vi "Begin.vi"(11 "Image Size":T1=enum."160x120") -> (0 "error out":errorcluster)   [LabVIEW 2012]
doc: "Called before other user functions, this VI is expected to open initial I/O refnums, load in file data, and do all program initialization. Notice that the <B>error out</B> terminal is simply used for data flow. Wiring it to other structures or subVIs ensures that this VI runs first."
uses:
  <vilib>/Rock Robotics/WPI/Camera/WPI_CameraImageSize.ctl
  <vilib>/Rock Robotics/WPI/SafetyOutput/WPI_SafetyOutputConfigMenu.ctl
  <vilib>/Rock Robotics/WPI/DriverStation/WPI_DriverStationRobotMode2.ctl
  <vilib>/Rock Robotics/WPI/Joystick/WPI_JoystickDeviceEnum.ctl
  <vilib>/Rock Robotics/SystemInterfaces/DIO/FPGA_DIOPWMChannel.ctl
  <vilib>/Rock Robotics/WPI/Solenoid/WPI_SolenoidChannel.ctl
  <vilib>/Rock Robotics/SystemInterfaces/DIO/FPGA_DIOChannel.ctl
  <vilib>/Rock Robotics/SystemInterfaces/DIO/FPGA_DIORelayChannel.ctl
  <vilib>/Rock Robotics/SystemInterfaces/AI/FPGA_AIChannel.ctl
  Robot Global Data.vi
  <vilib>/Rock Robotics/WPI/MotorControl/WPI_MotorControlOpen Talon.vi
  <vilib>/Rock Robotics/WPI/RobotDrive/WPI_RobotDriveOpen4MotorWithTalon.vi
  <vilib>/Rock Robotics/WPI/Solenoid/WPI_SolenoidOpenDouble.vi
  <vilib>/Rock Robotics/WPI/MotorControl/WPI_MotorControlOpen Victor.vi
  <vilib>/Rock Robotics/WPI/Counter/WPI_CounterDigitalInputToDigitalSource.vi
  <vilib>/Rock Robotics/WPI/Compressor/WPI_CompressorGetSetRefNum.vi
  <vilib>/Rock Robotics/WPI/Camera/WPI_CameraWhite Balance Values.ctl
  <vilib>/Rock Robotics/WPI/Camera/WPI_CameraExposure Values.ctl
  <vilib>/Rock Robotics/WPI/Camera/WPI_CameraFrameRate.ctl
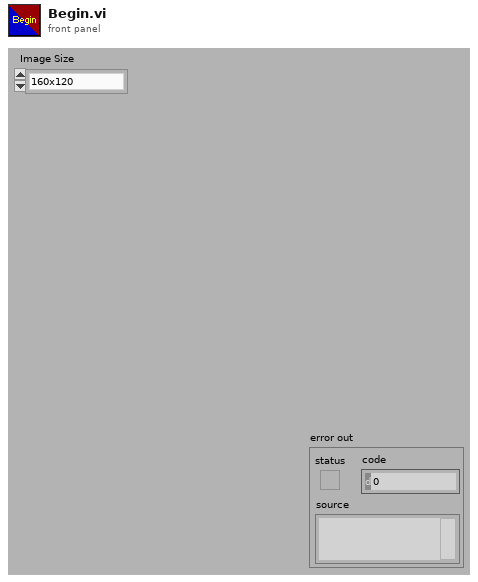
[diagram p1: front panel]
types:
  T1 = typedef "WPI_CameraImageSize.ctl" = enum16{"640x480", "320x240", "160x120"}
  T2 = typedef "FPGA_DIOChannel.ctl" = enum8{"DIO 1", "DIO 2", "DIO 3", "DIO 4", "DIO 5", "DIO 6", "DIO 7", "DIO 8", "DIO 9", "DIO 10", "DIO 11", "DIO 12", "DIO 13", "DIO 14", "Invalid"}
  T3 = typedef "WPI_SolenoidChannel.ctl" = enum8{"Solenoid 1", "Solenoid 2", "Solenoid 3", "Solenoid 4", "Solenoid 5", "Solenoid 6", "Solenoid 7", "Solenoid 8", "Invalid"}
  T4 = typedef "FPGA_AIChannel.ctl" = enum8{"AI 1", "AI 2", "AI 3", "AI 4", "AI 5", "AI 6", "AI 7", "AI 8", "Invalid"}
  T5 = typedef "FPGA_DIOPWMChannel.ctl" = enum8{"PWM 1", "PWM 2", "PWM 3", "PWM 4", "PWM 5", "PWM 6", "PWM 7", "PWM 8", "PWM 9", "PWM 10", "Invalid"}
  T6 = typedef "FPGA_DIORelayChannel.ctl" = enum8{"Relay 1", "Relay 2", "Relay 3", "Relay 4", "Relay 5", "Relay 6", "Relay 7", "Relay 8", "Invalid"}
  T7 = typedef "WPI_JoystickDeviceEnum.ctl" = enum16{"USB 1", "USB 2", "USB 3", "USB 4", "Kinect 1", "Kinect 2"}
  T8 = typedef "WPI_DriverStationRobotMode2.ctl" = enum16{"Autonomous Disabled", "Autonomous Enabled", "Teleop Disabled", "Teleop Enabled", "Timeout", "Finish", "Test Disabled", "Test Enabled"}
  T9 = typedef "WPI_SafetyOutputConfigMenu.ctl" = enum16{"Enable", "Disable"}
  T10 = typedef "WPI_CameraFrameRate.ctl" = u32
  T11 = typedef "WPI_CameraExposure Values.ctl" = enum16{"Auto", "Flicker-free 50 Hz", "Flicker-free 60 Hz", "Hold current"}
  T12 = typedef "WPI_CameraWhite Balance Values.ctl" = enum16{"Auto", "Fixed indoor", "Fixed outdoor 1", "Fixed outdoor 2", "Fixed fluorescent 1", "Fixed fluorescent 2", "Hold current"}
  T13 = typedef "WPI_CameraDevRef.ctl" = cluster{"Camera Address":string, "CameraStatus":errorcluster, "Acquire Image Notifier":refnum<notifier>}
  T14 = typedef "WPI_RobotDriveDevRef.ctl" = cluster{"DevStatus":errorcluster, "Motors[]":T15[], "Square Inputs":bool, "Max Output":dbl, "Isochronous":bool}
  T15 = typedef "WPI_MotorControlDeviceRef.ctl" = cluster{"DeviceStatus":errorcluster, "Type":enum16{"PWM", "CAN"}, "PWM":cluster{"Digital Module":T16, "PWM Channel":T5, "DeadBand":T17}, "CAN":cluster{"Device Number":u8, "Control Mode":T18, "Semaphore":T19, "Max Vout":dbl}, "Invert":bool, "TransformRef":T20, "InvTransformRef":T20}
  T16 = typedef "FPGA_TypedefDigitalModule.ctl" = enum16{"Digital Module 1", "Digital Module 2"}
  T17 = typedef "WPI_PWMDeadband.ctl" = cluster{"Name":string, "maxPositivePwm":i32, "minPositivePwm":i32, "centerPwm":i32, "maxNegativePwm":i32, "minNegativePwm":i32, "angularRange":u16}
  T18 = typedef "WPI_CANJaguar_ControlMode.ctl" = enum8{"Percent VBus", "Current", "Speed", "Position", "Voltage"}
  T19 = typedef "Semaphore RefNum" = refnum<k1>
  T20 = typedef "WPI_PWMTransform_ConPane.ctl" = refnum<vi>
  T21 = typedef "WPI_DigitalInputDevRef.ctl" = cluster{"DevStatus":errorcluster, "DIO Channel":T2, "Digital Module":T16}
  T22 = typedef "WPI_SolenoidDevRef.ctl" = cluster{"DevStatus":errorcluster, "Solenoid Module":T23, "Forward Solenoid Channel":T3, "Reverse Solenoid Channel":T3}
  T23 = typedef "FPGA_TypedefSolenoidModule.ctl" = enum16{"Solenoid Module 1", "Solenoid Module 2"}
  T24 = typedef "WPI_CompressorDevRef.ctl" = cluster{"DevStatus":errorcluster, "DigitalInputDevRef":T21, "RelayDevRef":T25}
  T25 = typedef "WPI_RelayDevRef.ctl" = cluster{"DevStatus":errorcluster, "Relay Channel":T6, "Digital Module":T16, "Relay Direction":T26}
  T26 = typedef "WPI_RelayDirection.ctl" = enum16{"Both directions", "Forward only", "Reverse only"}
  T27 = typedef "WPI_JoystickDevRef.ctl" = cluster{"Device":T7}
  T28 = typedef "WPI_AnalogChannelDevRef.ctl" = cluster{"DevStatus":errorcluster, "Analog Module":T29, "Analog Channel":T4}
  T29 = typedef "FPGA_TypedefAnalogModule.ctl" = enum16{"Analog Module 1", "Analog Module 2"}
  T30 = typedef "FPGA_CounterEncoderSourceConvertionLVSourceType.ctl" = cluster{"DevStatus":errorcluster, "AnalogTriggerMode?":bool, "DigitalMode":cluster{"Digital Module":T16, "DIO Channel":T31}, "AnalogTriggerMode":cluster{"AnalogTriggerIndex":T32, "OutputType":T33}}
  T31 = typedef "FPGA_DIODigitalSourceChannel.ctl" = enum8{"DIO 1", "DIO 2", "DIO 3", "DIO 4", "DIO 5", "DIO 6", "DIO 7", "DIO 8", "DIO 9", "DIO 10", "DIO 11", "DIO 12", "DIO 13", "DIO 14", "Disabled"}
  T32 = typedef "FPGA_AnalogTriggerIndex.ctl" = enum8{"Trig 0", "Trig 1", "Trig 2", "Trig 3", "Trig 4", "Trig 5", "Trig 6", "Trig 7", "Invalid"}
  T33 = typedef "FPGA_AnalogTriggerOutType.ctl" = enum16{"InWindow", "TriggerState", "Rising", "Falling"}
  T34 = typedef "WPI_EncoderDevRef.ctl" = cluster{"DevStatus":errorcluster, "EncoderIndex":T35, "CounterIndex":T36, "DistancePerCount":dbl, "Decoding Type":T37}
  T35 = typedef "FPGA_EncoderIdx.ctl" = enum8{"Enc 0", "Enc 1", "Enc 2", "Enc 3", "Invalid"}
  T36 = typedef "FPGA_CounterCtrSystemIndex.ctl" = enum8{"Ctr 0", "Ctr 1", "Ctr 2", "Ctr 3", "Ctr 4", "Ctr 5", "Ctr 6", "Ctr 7", "Invalid"}
  T37 = typedef "WPI_EncoderType.ctl" = enum16{"1x", "2x", "4x"}
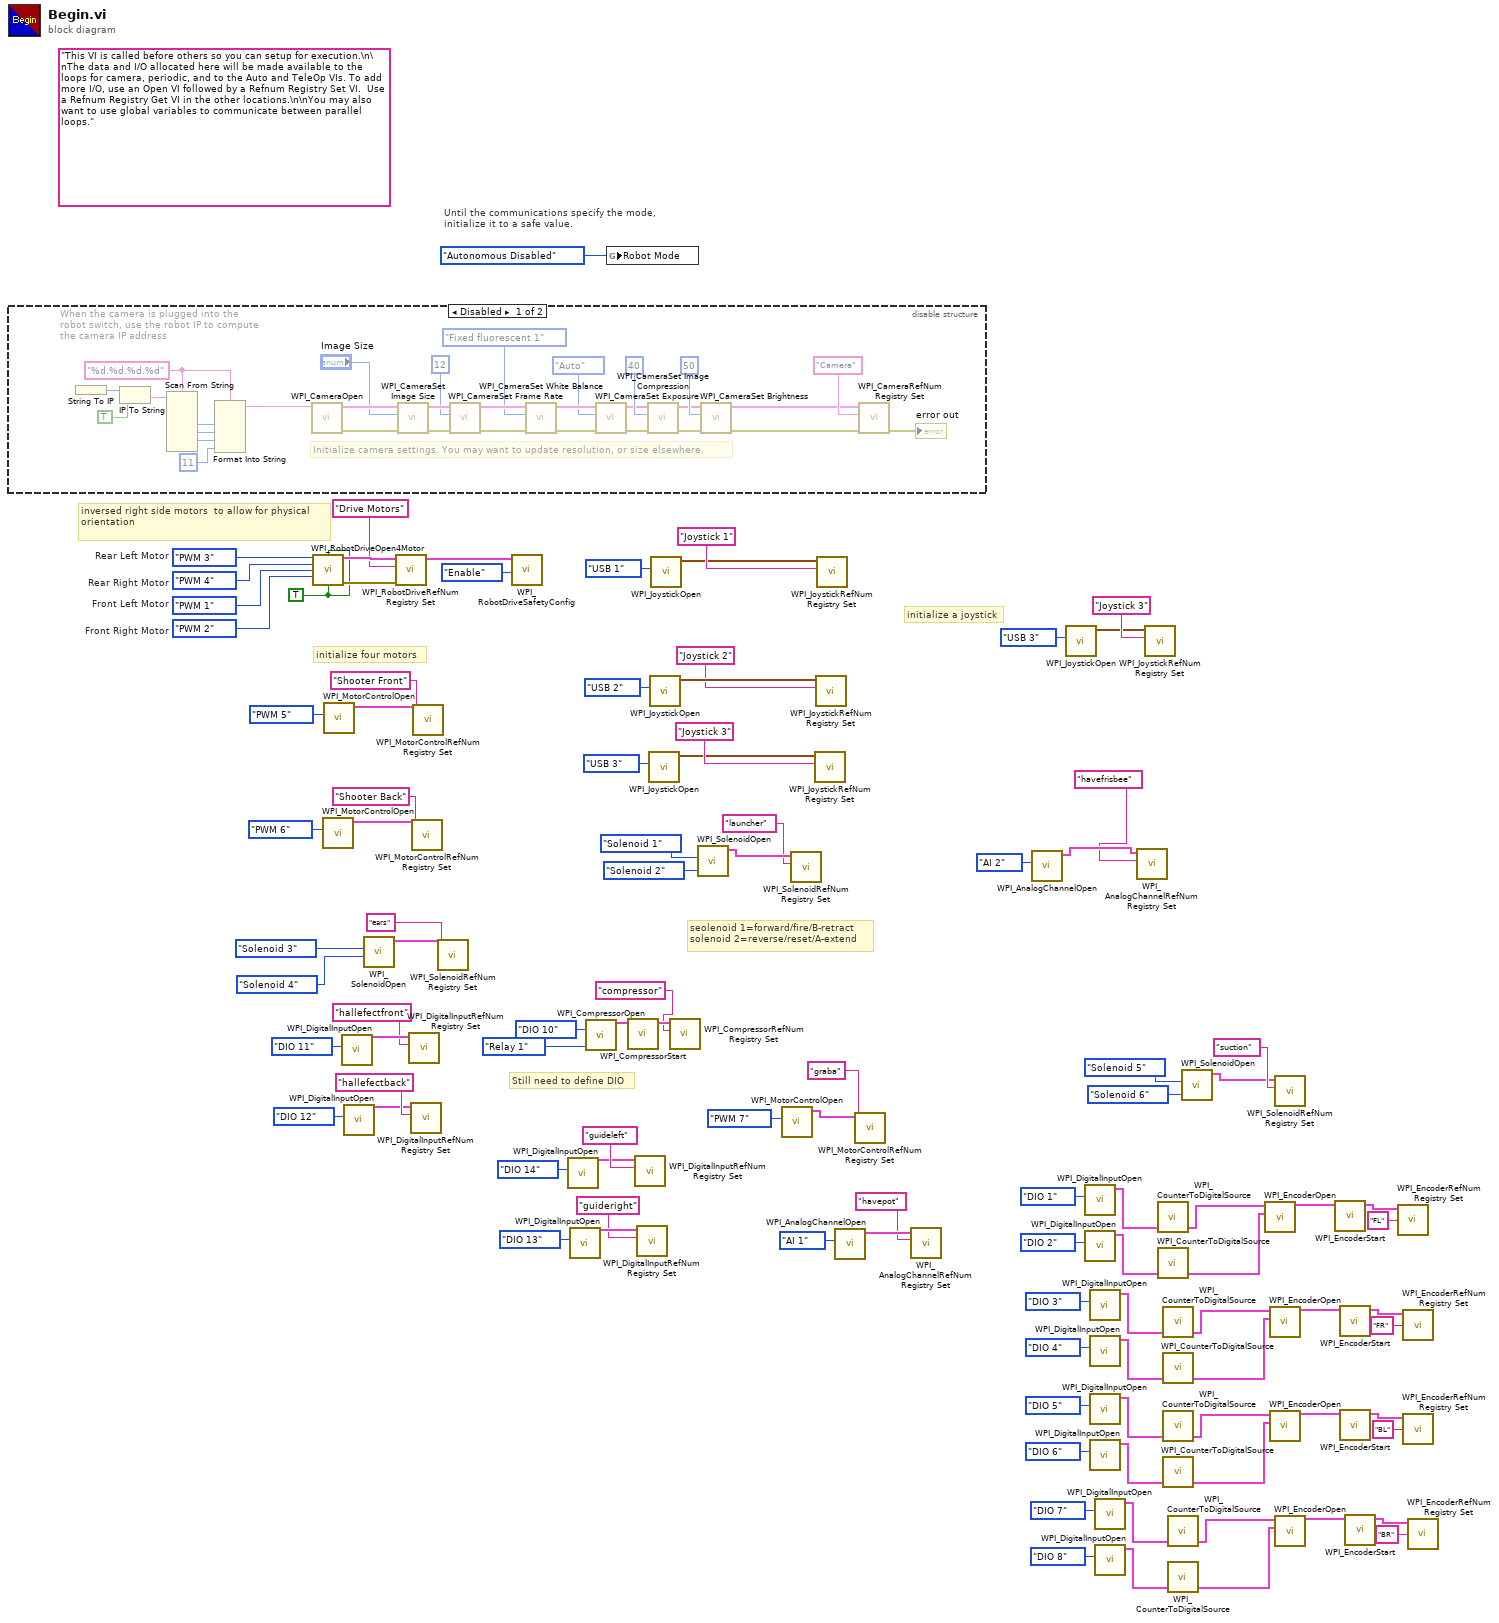
[diagram p0: block diagram]
diagram:
  w84 = TRUE ("Front Right Motor Inverted")
  w91 = FPGA_DIOPWMChannel."PWM 2"  # Front Right Motor
  w92 = FPGA_DIOPWMChannel."PWM 1"  # Front Left Motor
  w93 = FPGA_DIOPWMChannel."PWM 4"  # Rear Right Motor
  w94 = FPGA_DIOPWMChannel."PWM 3"  # Rear Left Motor
  (unwired) "This VI is called before others so you can setup for execution.\n\nThe data and I/O allocated here will be made available to the loops for camera, periodic, and to the Auto and TeleOp VIs. To add more I/O, use an Open VI followed by a Refnum Registry Set VI.  Use a Refnum Registry Get VI in the other locations.\n\nYou may also want to use global variables to communicate between parallel loops."
  # "Still need to define DIO"
  # "seolenoid 1=forward/fire/B-retract\nsolenoid 2=reverse/reset/A-extend"
  # "initialize a joystick"
  # "inversed right side motors  to allow for physical orientation"
  # "Until the communications specify the mode,\ninitialize it to a safe value."
  # "initialize four motors"
  n1 = disable-structure shown="Disabled" {
    frame Disabled {
      w106 = "%d.%d.%d.%d" ("format string")
      # "When the camera is plugged into the\nrobot switch, use the robot IP to compute\nthe camera IP address"
      # "Initialize camera settings. You may want to update resolution, or size elsewhere."
      n2 = String To IP() -> (0:w113:u32)  [unwired: 1 in]
      n3 = IP To String(1:TRUE ("dot notation? (F)"), 2:w113) -> (0:w111:string)
      n4 = Scan From String(format string=w106, input string=w111) -> (output 1=w110:i32, output 2=w109:i32, output 3=w108:i32)  [unwired: 7 in, 3 out]
      n5 = Format Into String(format string=w106, w110, w109, w108, 11 ("Compression")) -> (resulting string=w105:string)  [unwired: 2 in, 1 out]
      n6 = call <vilib>:"WPI_CameraOpen.vi"("Camera Address"=w105) -> ("error out"=w125:errorcluster, "CameraDevRef"=w126:T13)  [unwired: 1 in, 8 out]
      n7 = call <vilib>:"WPI_CameraSet Image Size.vi"("error in (no error)"=w125, "Image Size"="Image Size", "CameraDevRef"=w126) -> ("error out"=w124:errorcluster, "CameraDevRef Out"=w127:T13)  [unwired: 7 out]
      n8 = call <vilib>:"WPI_CameraSet Frame Rate.vi"("error in (no error)"=w124, "Frame Rate (fps)"=T10 12, "CameraDevRef"=w127) -> ("error out"=w123:errorcluster, "CameraDevRef Out"=w129:T13)  [unwired: 7 out]
      n9 = call <vilib>:"WPI_CameraSet White Balance.vi"("error in (no error)"=w123, "White Balance"=WPI_CameraWhite_Balance_Values."Fixed fluorescent 1", "CameraDevRef"=w129) -> ("error out"=w122:errorcluster, "CameraDevRef Out"=w128:T13)  [unwired: 7 out]
      n10 = call <vilib>:"WPI_CameraSet Exposure.vi"("error in (no error)"=w122, "Exposure"=WPI_CameraExposure_Values."Auto", "CameraDevRef"=w128) -> ("error out"=w121:errorcluster, "CameraDevRef Out"=w131:T13)  [unwired: 7 out]
      n11 = call <vilib>:"WPI_CameraSet Image Compression.vi"("error in (no error)"=w121, "Compression"=40, "CameraDevRef"=w131) -> ("error out"=w120:errorcluster, "CameraDevRef Out"=w130:T13)  [unwired: 7 out]
      n12 = call <vilib>:"WPI_CameraSet Brightness.vi"("error in (no error)"=w120, "Brightness"=50, "CameraDevRef"=w130) -> ("error out"=w118:errorcluster, "CameraDevRef Out"=w119:T13)  [unwired: 7 out]
      n13 = call <vilib>:"WPI_CameraRefNum Registry Set.vi"("error in (no error)"=w118, "refnum name"="Camera", "CameraDevRef"=w119) -> ("error out"=→"error out":errorcluster)  [unwired: 8 out]
    }
    frame Enabled {
    }
  }
  n14 = call-poly <vilib>:"WPI_RobotDriveOpen4Motor.vi"("Rear Left Motor"=w94, "Rear Right Motor Inverted"=w84, "Rear Right Motor"=w93, "Front Left Motor"=w92, "Front Right Motor"=w91, "Front Right Motor Inverted"=w84) -> ("RobotDriveDevRef"=w103:T14, "error out"=w101:errorcluster)  [unwired: 8 in]
  n15 = call-poly <vilib>:"WPI_MotorControlOpen.vi"("PWM Channel"=FPGA_DIOPWMChannel."PWM 6") -> ("MotorControlDeviceRef"=w78:T15)  [unwired: 9 in, 1 out]
  n16 = call-poly <vilib>:"WPI_MotorControlOpen.vi"("PWM Channel"=FPGA_DIOPWMChannel."PWM 5") -> ("MotorControlDeviceRef"=w87:T15)  [unwired: 9 in, 1 out]
  n17 = call <vilib>:"WPI_DigitalInputOpen.vi"("DIO Channel"=FPGA_DIOChannel."DIO 11") -> ("DigitalInputDevRef"=w61:T21)  [unwired: 9 in, 1 out]
  n18 = call <vilib>:"WPI_DigitalInputOpen.vi"("DIO Channel"=FPGA_DIOChannel."DIO 12") -> ("DigitalInputDevRef"=w56:T21)  [unwired: 9 in, 1 out]
  n19 = call-poly <vilib>:"WPI_SolenoidOpen.vi"("Reverse Solenoid Channel"=WPI_SolenoidChannel."Solenoid 4", "Forward Solenoid Channel"=WPI_SolenoidChannel."Solenoid 3" ("Reverse Solenoid Channel")) -> ("SolenoidDevRef"=w68:T22)  [unwired: 8 in, 1 out]
  n20 = call <vilib>:"WPI_RobotDriveRefNum Registry Set.vi"("error in (no error)"=w101, "refnum name"="Drive Motors", "RobotDriveDevRef"=w103) -> ("RobotDriveDevRef"=w100:T14)  [unwired: 8 out]
  n21 = call <vilib>:"WPI_DigitalInputRefNum Registry Set.vi"("refnum name"="hallefectfront", "DigitalInputDevRef"=w61) -> ()  [unwired: 8 in, 2 out]
  n22 = call <vilib>:"WPI_DigitalInputRefNum Registry Set.vi"("refnum name"="hallefectback", "DigitalInputDevRef"=w56) -> ()  [unwired: 8 in, 2 out]
  n23 = call <vilib>:"WPI_MotorControlRefNum Registry Set.vi"("refnum name"="Shooter Back", "MotorControlDevRef"=w78) -> ()  [unwired: 8 in, 2 out]
  n24 = call <vilib>:"WPI_MotorControlRefNum Registry Set.vi"("refnum name"="Shooter Front", "MotorControlDevRef"=w87) -> ()  [unwired: 8 in, 2 out]
  n25 = call <vilib>:"WPI_SolenoidRefNum Registry Set.vi"("refnum name"="ears", "SolenoidDevRef"=w68) -> ()  [unwired: 8 in, 2 out]
  n26 = call <vilib>:"WPI_RobotDriveSafetyConfig.vi"("mode"=WPI_SafetyOutputConfigMenu."Enable", "RobotDriveDevRef"=w100) -> ()  [unwired: 8 in, 2 out]
  n27 = call <vilib>:"WPI_DigitalInputOpen.vi"("DIO Channel"=FPGA_DIOChannel."DIO 14") -> ("DigitalInputDevRef"=w50:T21)  [unwired: 9 in, 1 out]
  n28 = call <vilib>:"WPI_DigitalInputOpen.vi"("DIO Channel"=FPGA_DIOChannel."DIO 13") -> ("DigitalInputDevRef"=w55:T21)  [unwired: 9 in, 1 out]
  n29 = call <vilib>:"WPI_CompressorOpen.vi"("Pressure Switch DIO Channel"=FPGA_DIOChannel."DIO 10", "Relay Channel"=FPGA_DIORelayChannel."Relay 1") -> ("CompressorDevRef"=w66:T24)  [unwired: 12 in, 1 out]
  n30 = global write "Robot Global Data.vi" "Robot Mode"(WPI_DriverStationRobotMode2."Autonomous Disabled" ("Robot Mode")) -> ()
  n31 = call <vilib>:"WPI_CompressorStart.vi"("CompressorDevRef"=w66) -> ("CompressorDevRef"=w65:T24)  [unwired: 9 in, 1 out]
  n32 = call <vilib>:"WPI_DigitalInputRefNum Registry Set.vi"("refnum name"="guideleft", "DigitalInputDevRef"=w50) -> ()  [unwired: 8 in, 2 out]
  n33 = call <vilib>:"WPI_DigitalInputRefNum Registry Set.vi"("refnum name"="guideright", "DigitalInputDevRef"=w55) -> ()  [unwired: 8 in, 2 out]
  n34 = call <vilib>:"WPI_JoystickOpen.vi"("JoystickDevice"=WPI_JoystickDeviceEnum."USB 3") -> ("JoystickDevRef"=w72:T27)  [unwired: 10 in]
  n35 = call <vilib>:"WPI_JoystickOpen.vi"("JoystickDevice"=WPI_JoystickDeviceEnum."USB 2") -> ("JoystickDevRef"=w89:T27)  [unwired: 10 in]
  n36 = call <vilib>:"WPI_JoystickOpen.vi"("JoystickDevice"=WPI_JoystickDeviceEnum."USB 1") -> ("JoystickDevRef"=w96:T27)  [unwired: 10 in]
  n37 = call <vilib>:"WPI_CompressorRefNum Registry Set.vi"("refnum name"="compressor", "CompressorDevRef"=w65) -> ()  [unwired: 8 in, 2 out]
  n38 = call-poly <vilib>:"WPI_SolenoidOpen.vi"("Reverse Solenoid Channel"=WPI_SolenoidChannel."Solenoid 2", "Forward Solenoid Channel"=WPI_SolenoidChannel."Solenoid 1") -> ("SolenoidDevRef"=w77:T22)  [unwired: 8 in, 1 out]
  n39 = call-poly <vilib>:"WPI_MotorControlOpen.vi"("PWM Channel"=FPGA_DIOPWMChannel."PWM 7") -> ("MotorControlDeviceRef"=w46:T15)  [unwired: 9 in, 1 out]
  n40 = call <vilib>:"WPI_SolenoidRefNum Registry Set.vi"("refnum name"="launcher", "SolenoidDevRef"=w77) -> ()  [unwired: 8 in, 2 out]
  n41 = call <vilib>:"WPI_JoystickRefNum Registry Set.vi"("refnum name"="Joystick 3", "JoystickDevRef"=w72) -> ()  [unwired: 8 in, 2 out]
  n42 = call <vilib>:"WPI_JoystickRefNum Registry Set.vi"("refnum name"="Joystick 2", "JoystickDevRef"=w89) -> ()  [unwired: 8 in, 2 out]
  n43 = call <vilib>:"WPI_JoystickRefNum Registry Set.vi"("refnum name"="Joystick 1", "JoystickDevRef"=w96) -> ()  [unwired: 8 in, 2 out]
  n44 = call <vilib>:"WPI_AnalogChannelOpen.vi"("Analog Channel"=FPGA_AIChannel."AI 1") -> ("AIDeviceRef"=w43:T28)  [unwired: 9 in, 1 out]
  n45 = call <vilib>:"WPI_MotorControlRefNum Registry Set.vi"("refnum name"="graba", "MotorControlDevRef"=w46) -> ()  [unwired: 8 in, 2 out]
  n46 = call <vilib>:"WPI_AnalogChannelRefNum Registry Set.vi"("refnum name"="havepot", "AIDeviceRef"=w43) -> ()  [unwired: 8 in, 2 out]
  n47 = call <vilib>:"WPI_AnalogChannelOpen.vi"("Analog Channel"=FPGA_AIChannel."AI 2") -> ("AIDeviceRef"=w49:T28)  [unwired: 9 in, 1 out]
  n48 = call <vilib>:"WPI_JoystickOpen.vi"("JoystickDevice"=WPI_JoystickDeviceEnum."USB 3") -> ("JoystickDevRef"=w82:T27)  [unwired: 10 in]
  n49 = call <vilib>:"WPI_DigitalInputOpen.vi"("DIO Channel"=FPGA_DIOChannel."DIO 1") -> ("DigitalInputDevRef"=w33:T21)  [unwired: 9 in, 1 out]
  n50 = call <vilib>:"WPI_DigitalInputOpen.vi"("DIO Channel"=FPGA_DIOChannel."DIO 2") -> ("DigitalInputDevRef"=w29:T21)  [unwired: 9 in, 1 out]
  n51 = call <vilib>:"WPI_DigitalInputOpen.vi"("DIO Channel"=FPGA_DIOChannel."DIO 3") -> ("DigitalInputDevRef"=w22:T21)  [unwired: 9 in, 1 out]
  n52 = call <vilib>:"WPI_DigitalInputOpen.vi"("DIO Channel"=FPGA_DIOChannel."DIO 4") -> ("DigitalInputDevRef"=w26:T21)  [unwired: 9 in, 1 out]
  n53 = call <vilib>:"WPI_DigitalInputOpen.vi"("DIO Channel"=FPGA_DIOChannel."DIO 5") -> ("DigitalInputDevRef"=w4:T21)  [unwired: 9 in, 1 out]
  n54 = call <vilib>:"WPI_DigitalInputOpen.vi"("DIO Channel"=FPGA_DIOChannel."DIO 6") -> ("DigitalInputDevRef"=w8:T21)  [unwired: 9 in, 1 out]
  n55 = call <vilib>:"WPI_DigitalInputOpen.vi"("DIO Channel"=FPGA_DIOChannel."DIO 7") -> ("DigitalInputDevRef"=w15:T21)  [unwired: 9 in, 1 out]
  n56 = call <vilib>:"WPI_DigitalInputOpen.vi"("DIO Channel"=FPGA_DIOChannel."DIO 8") -> ("DigitalInputDevRef"=w11:T21)  [unwired: 9 in, 1 out]
  n57 = call <vilib>:"WPI_AnalogChannelRefNum Registry Set.vi"("refnum name"="havefrisbee", "AIDeviceRef"=w49) -> ()  [unwired: 8 in, 2 out]
  n58 = call <vilib>:"WPI_JoystickRefNum Registry Set.vi"("refnum name"="Joystick 3", "JoystickDevRef"=w82) -> ()  [unwired: 8 in, 2 out]
  n59 = call-poly <vilib>:"WPI_CounterToDigitalSource.vi"("DigitalInputDevRef"=w33) -> ("Digital Source"=w32:T30)  [unwired: 6 in]
  n60 = call-poly <vilib>:"WPI_CounterToDigitalSource.vi"("DigitalInputDevRef"=w29) -> ("Digital Source"=w28:T30)  [unwired: 6 in]
  n61 = call-poly <vilib>:"WPI_CounterToDigitalSource.vi"("DigitalInputDevRef"=w22) -> ("Digital Source"=w23:T30)  [unwired: 6 in]
  n62 = call-poly <vilib>:"WPI_CounterToDigitalSource.vi"("DigitalInputDevRef"=w26) -> ("Digital Source"=w27:T30)  [unwired: 6 in]
  n63 = call-poly <vilib>:"WPI_CounterToDigitalSource.vi"("DigitalInputDevRef"=w4) -> ("Digital Source"=w5:T30)  [unwired: 6 in]
  n64 = call-poly <vilib>:"WPI_CounterToDigitalSource.vi"("DigitalInputDevRef"=w8) -> ("Digital Source"=w9:T30)  [unwired: 6 in]
  n65 = call-poly <vilib>:"WPI_CounterToDigitalSource.vi"("DigitalInputDevRef"=w15) -> ("Digital Source"=w14:T30)  [unwired: 6 in]
  n66 = call-poly <vilib>:"WPI_CounterToDigitalSource.vi"("DigitalInputDevRef"=w11) -> ("Digital Source"=w10:T30)  [unwired: 6 in]
  n67 = call-poly <vilib>:"WPI_SolenoidOpen.vi"("Reverse Solenoid Channel"=WPI_SolenoidChannel."Solenoid 6", "Forward Solenoid Channel"=WPI_SolenoidChannel."Solenoid 5") -> ("SolenoidDevRef"=w37:T22)  [unwired: 8 in, 1 out]
  n68 = call <vilib>:"WPI_EncoderOpen.vi"("BSource"=w28, "ASource"=w32) -> ("EncoderDevRef"=w36:T34)  [unwired: 8 in, 1 out]
  n69 = call <vilib>:"WPI_EncoderOpen.vi"("BSource"=w27, "ASource"=w23) -> ("EncoderDevRef"=w19:T34)  [unwired: 8 in, 1 out]
  n70 = call <vilib>:"WPI_EncoderOpen.vi"("BSource"=w9, "ASource"=w5) -> ("EncoderDevRef"=w1:T34)  [unwired: 8 in, 1 out]
  n71 = call <vilib>:"WPI_SolenoidRefNum Registry Set.vi"("refnum name"="suction", "SolenoidDevRef"=w37) -> ()  [unwired: 8 in, 2 out]
  n72 = call <vilib>:"WPI_EncoderOpen.vi"("BSource"=w10, "ASource"=w14) -> ("EncoderDevRef"=w18:T34)  [unwired: 8 in, 1 out]
  n73 = call <vilib>:"WPI_EncoderStart.vi"("EncoderDevRef"=w36) -> ("EncoderDevRef"=w35:T34)  [unwired: 9 in, 1 out]
  n74 = call <vilib>:"WPI_EncoderStart.vi"("EncoderDevRef"=w19) -> ("EncoderDevRef"=w20:T34)  [unwired: 9 in, 1 out]
  n75 = call <vilib>:"WPI_EncoderStart.vi"("EncoderDevRef"=w1) -> ("EncoderDevRef"=w2:T34)  [unwired: 9 in, 1 out]
  n76 = call <vilib>:"WPI_EncoderStart.vi"("EncoderDevRef"=w18) -> ("EncoderDevRef"=w17:T34)  [unwired: 9 in, 1 out]
  n77 = call <vilib>:"WPI_EncoderRefNum Registry Set.vi"("refnum name"="FL", "EncoderDevRef"=w35) -> ()  [unwired: 8 in, 2 out]
  n78 = call <vilib>:"WPI_EncoderRefNum Registry Set.vi"("refnum name"="FR", "EncoderDevRef"=w20) -> ()  [unwired: 8 in, 2 out]
  n79 = call <vilib>:"WPI_EncoderRefNum Registry Set.vi"("refnum name"="BL", "EncoderDevRef"=w2) -> ()  [unwired: 8 in, 2 out]
  n80 = call <vilib>:"WPI_EncoderRefNum Registry Set.vi"("refnum name"="BR", "EncoderDevRef"=w17) -> ()  [unwired: 8 in, 2 out]
